vi "List Headers.vi"(8 "error in":errorcluster, 11 "session in":refnum<class "Session.lvclass">) -> (0 "error out":errorcluster, 2 "headers":string, 3 "session out":refnum<class "Session.lvclass">)   [LabVIEW 2020, in "Library Commun.lvlib" / "Library Http.lvlib" / "Session.lvclass"]
doc: "Lists the headers associated with the HTTP session. Headers define attributes of the data exchanged between the client and server."
uses:
  Session.lvclass
  Session.lvclass/Session.ctl
  lvwebclient_32.dll
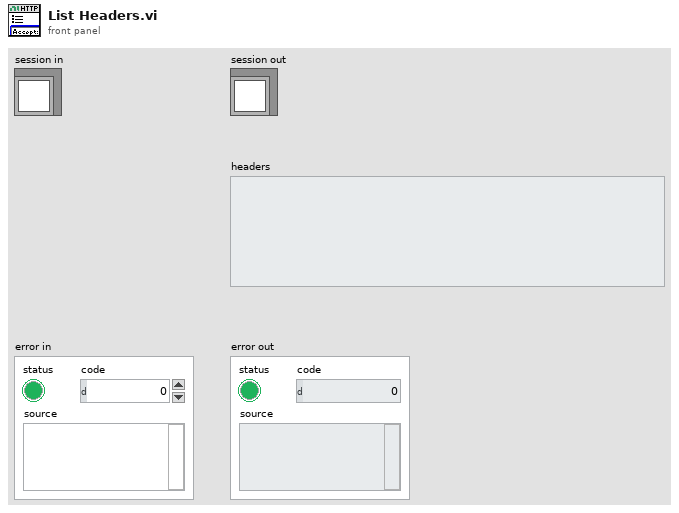
[diagram p1: front panel]
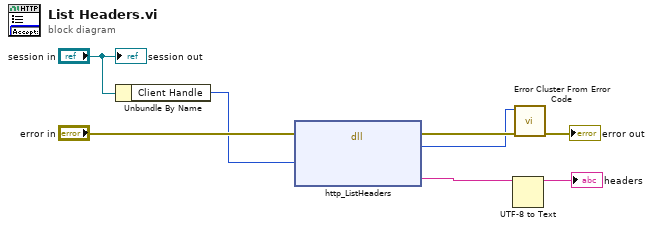
[diagram p0: block diagram]
diagram:
  n1 = Unbundle By Name("session in") -> ("Client Handle"=w2:u32)
  n2 = dll-call lib="C:/Users/ngarcin/OneDrive - Altyor/Standard TB/Class/Http Altyor/lvwebclient_*.*" fn="http_ListHeaders"(error in="error in", "handle"=w2) -> (error out=w4:errorcluster, "return"=w3:i32, "resultHeader"=w1:string)  [unwired: 4 in, 1 out]
  n3 = UTF-8 to Text(11:w1) -> (3:→"headers":string)  [unwired: 2 in, 1 out]
  n4 = call <vilib>:"Error Cluster From Error Code.vi"("error in (no error)"=w4, "error code (0)"=w3) -> ("error out"=→"error out":errorcluster)  [unwired: 7 in]
  "session out" <- "session in"
